vi "DataFilePath _ Write INI File.vi"(6 "AutoInterval":i32 caption="自动挑点时间间隔：", 7 "FileNote":string="FileName", 8 "error in":errorcluster, 9 "FileName":string="FileName", 10 "DataFolder":path, 11 "INI File":path) -> (0 "error out":errorcluster)   [LabVIEW 2016]
uses:
  <vilib>/Utility/config.llb/Write Key (Path).vi
  <vilib>/Utility/config.llb/Write Key (String).vi
  <vilib>/Utility/config.llb/Write Key (I32).vi
  <vilib>/Utility/config.llb/NI_LVConfig.lvlib
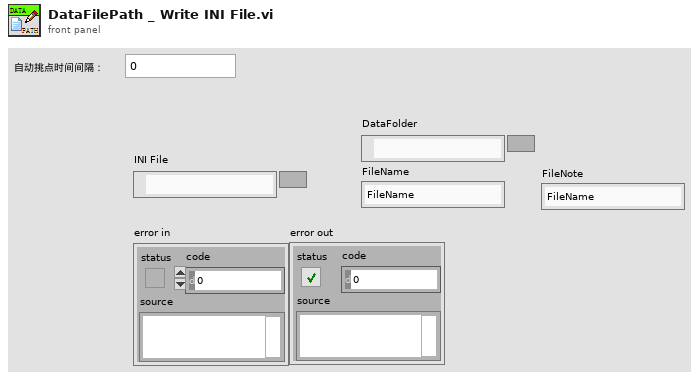
[diagram p1: front panel]
types:
  T1 = typedef "NI_LVConfig.lvlib/Config Data RefNum.ctl" = refnum<k1>
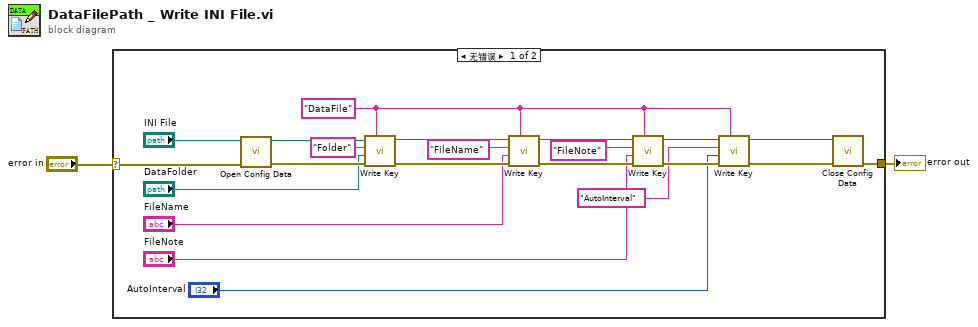
[diagram p0: block diagram]
diagram:
  n1 = case shown="无错误" "error in" {
    selector: "error in" -> [w13 w23]
    tunnel: [w12 w23] -> w1
    frame No Error {
      w5 = "DataFile" ("section")
      n2 = call <vilib>:"Open Config Data.vi"("error in (no error)"=w13, "configuration file path"="INI File") -> ("error out"=w21:errorcluster, "refnum"=w22:T1)  [unwired: 7 in, 1 out]
      n3 = call-poly <vilib>:"Write Key.vi"("section"=w5, "error in (no error)"=w21, "value"="DataFolder", "key"="Folder", "refnum"=w22) -> ("error out"=w19:errorcluster, "refnum out"=w18:T1)  [unwired: 4 in, 1 out]
      n4 = call-poly <vilib>:"Write Key.vi"("section"=w5, "error in (no error)"=w19, "value"="FileName", "key"="FileName", "refnum"=w18) -> ("error out"=w16:errorcluster, "refnum out"=w15:T1)  [unwired: 4 in, 1 out]
      n5 = call-poly <vilib>:"Write Key.vi"("section"=w5, "value"="FileNote", "key"="FileNote", "refnum"=w15) -> ("refnum out"=w9:T1)  [unwired: 5 in, 2 out]
      n6 = call-poly <vilib>:"Write Key.vi"("section"=w5, "value"="AutoInterval", "key"="AutoInterval", "refnum"=w9) -> ("refnum out"=w6:T1)  [unwired: 5 in, 2 out]
      n7 = call <vilib>:"Close Config Data.vi"("error in (no error)"=w16, "refnum"=w6) -> ("error out"=w12:errorcluster)  [unwired: 8 in, 1 out]
    }
    frame Error {
    }
  }
  "error out" <- w1
